vi "Acquisizione statica.vi"() -> ()   [LabVIEW 2017]
uses:
  <vilib>/Analysis/4window.llb/windowTd.ctl
  <vilib>/measure/maspectr.llb/Power Spectrum and PSD Export Mode.ctl
  <vilib>/DAQmx/read.llb/DAQmx Read (Analog 1D Wfm NChan NSamp).vi
  <vilib>/DAQmx/configure/timing.llb/DAQmx Timing (Sample Clock).vi
  <vilib>/DAQmx/miscellaneous.llb/DAQmx Fill In Error Info.vi
  <vilib>/measure/maspectr.llb/FFT Power Spectrum and PSD for N Chan.vi
  <vilib>/measure/maspectr.llb/FFT Spectrum (Mag-Phase) for N Chan.vi
  <vilib>/measure/maspectr.llb/Frequency Response Function (Mag-Phase) N-M.vi
  <vilib>/Waveform/WDTOps.llb/WDT Index Channel DBL.vi
  <vilib>/Waveform/WDTOps.llb/WDT Append Waveforms DBL.vi
  <vilib>/measure/NI_MAPro.lvlib
  <vilib>/Analysis/NI_AALPro.lvlib
panel:
  out "iterazioni":i32
  out "out":bool
  out "error out":errorcluster
  out "salvato":bool
  out "std dev":bool
  out "mean":bool
  out "sample":i32
  in  "std dev max":dbl
  in  "mean/sample max":dbl
  out "mean/sample":dbl
  out "mean":dbl format="%0.2f"
  out "std dev/semple":dbl
  out "standard deviation":dbl format="%0.2f"
  in  "Massa":string="_"
  in  "secondi da salvare":i32=1
  in  "restart averaging (F)":bool
  in  "window":T1 items=["Rectangle"=0, "Hanning"=1, "Hamming"=2, "Blackman-Harris"=3, "Exact Blackman"=4, "Blackman"=5, "Flat Top"=6, "4 Term B-Harris "=7, "7 Term B-Harris"=8, "Low Sidelobe"=9, "Blackman Nuttall"=11, "Triangle"=30, "Bartlett-Hanning"=31, "Bohman"=32, "Parzen"=33, "Welch"=34, "Kaiser"=60, "Dolph-Chebyshev"=61, "Gaussian"=62]
  in  "averaging parameters":T2={"averaging mode"=enum."Vector averaging", "weighting mode"=enum."Linear", "number of averages"=1000}
  in  "Tab Control 2":enum32{"TH", "FRF", "PSD", "FFT"}(tab)
  out "Waveform Chart":waveform(dbl)[](graph)
  out "Waveform Graph":cluster{"f0":dbl, "df":dbl, "magnitude":dbl[]}[](graph)
  in  "REFERENCE CHANNEL":i32=1
  out "Waveform Graph 2":cluster{"f0":dbl, "df":dbl, "magnitude":dbl[]}[](graph)
  out "Magnitude 2":cluster{"f0":dbl, "df":dbl, "magnitude":dbl[]}[](graph)
  out "Magnitude":cluster{"f0":dbl, "df":dbl, "magnitude":dbl[]}[](graph)
  in  "SAVE?":bool
  in  "export":path
  in  "stop":bool
  in  "acquisition":T3={"Fs"=2000.0, "group sample/s"=2000, "generation task"="ModAnalEs"} {"Fs" format="%.2p"}
  # "x10^-3"
  # "x10^-6"
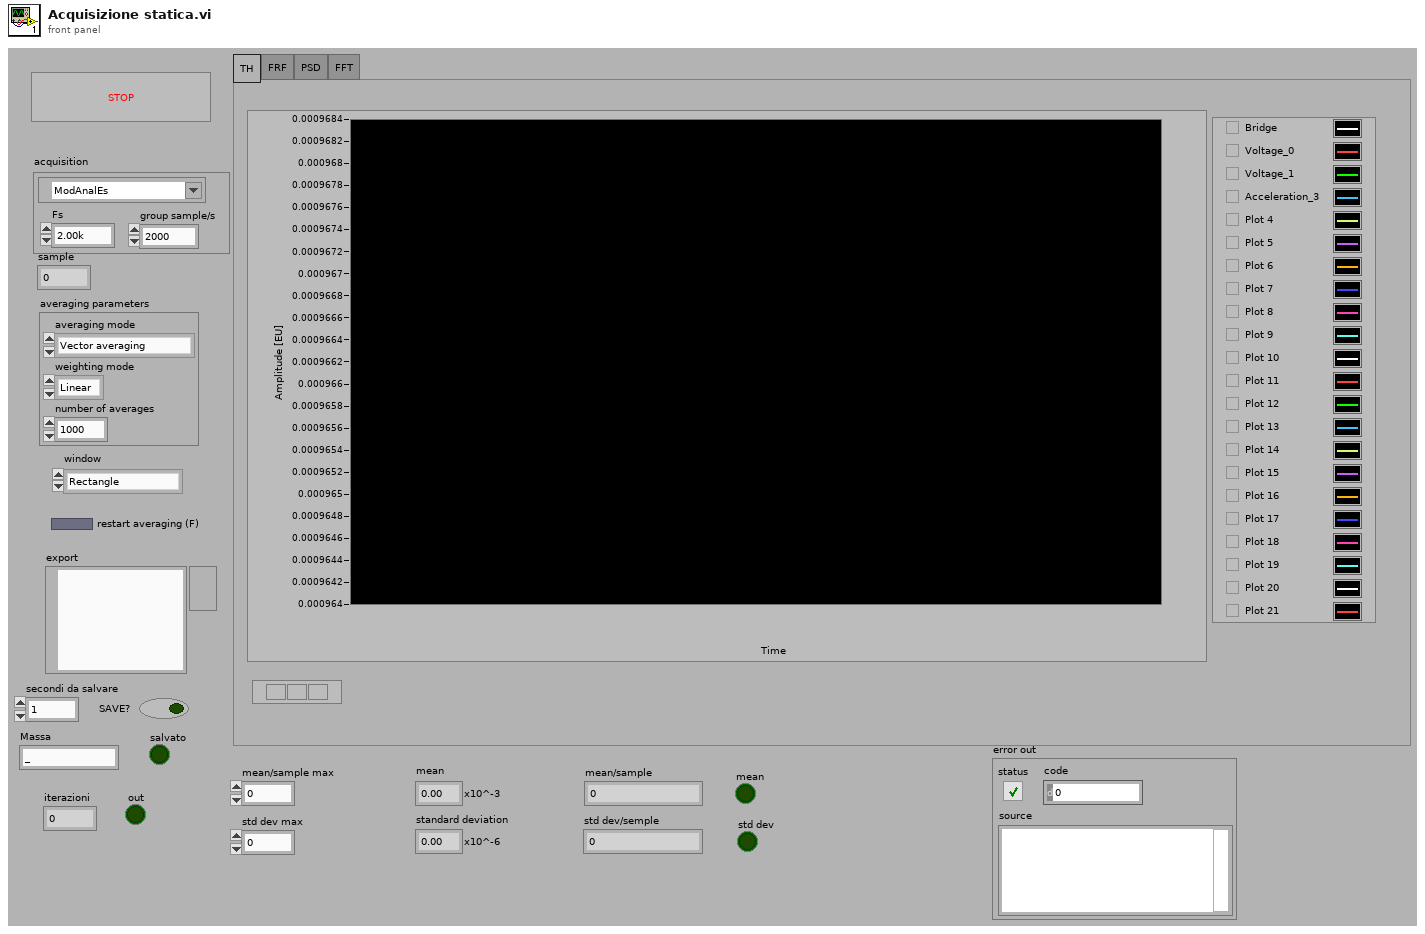
[diagram p1: front panel]
types:
  T1 = typedef "NI_AALPro.lvlib/windowTd.ctl" = u32
  T2 = cluster{"averaging mode":enum16{"No averaging", "Vector averaging", "RMS averaging", "Peak hold"}, "weighting mode":enum16{"Linear", "Exponential"}, "number of averages":u32}
  T3 = cluster{"Fs":dbl, "group sample/s":i32, "generation task":refnum<k21>}
  T4 = cluster{"dB On (F)":bool, "unwrap phase (F)":bool, "convert to degree (F)":bool}
  T5 = typedef "NI_MAPro.lvlib/Power Spectrum and PSD Export Mode.ctl" = u16
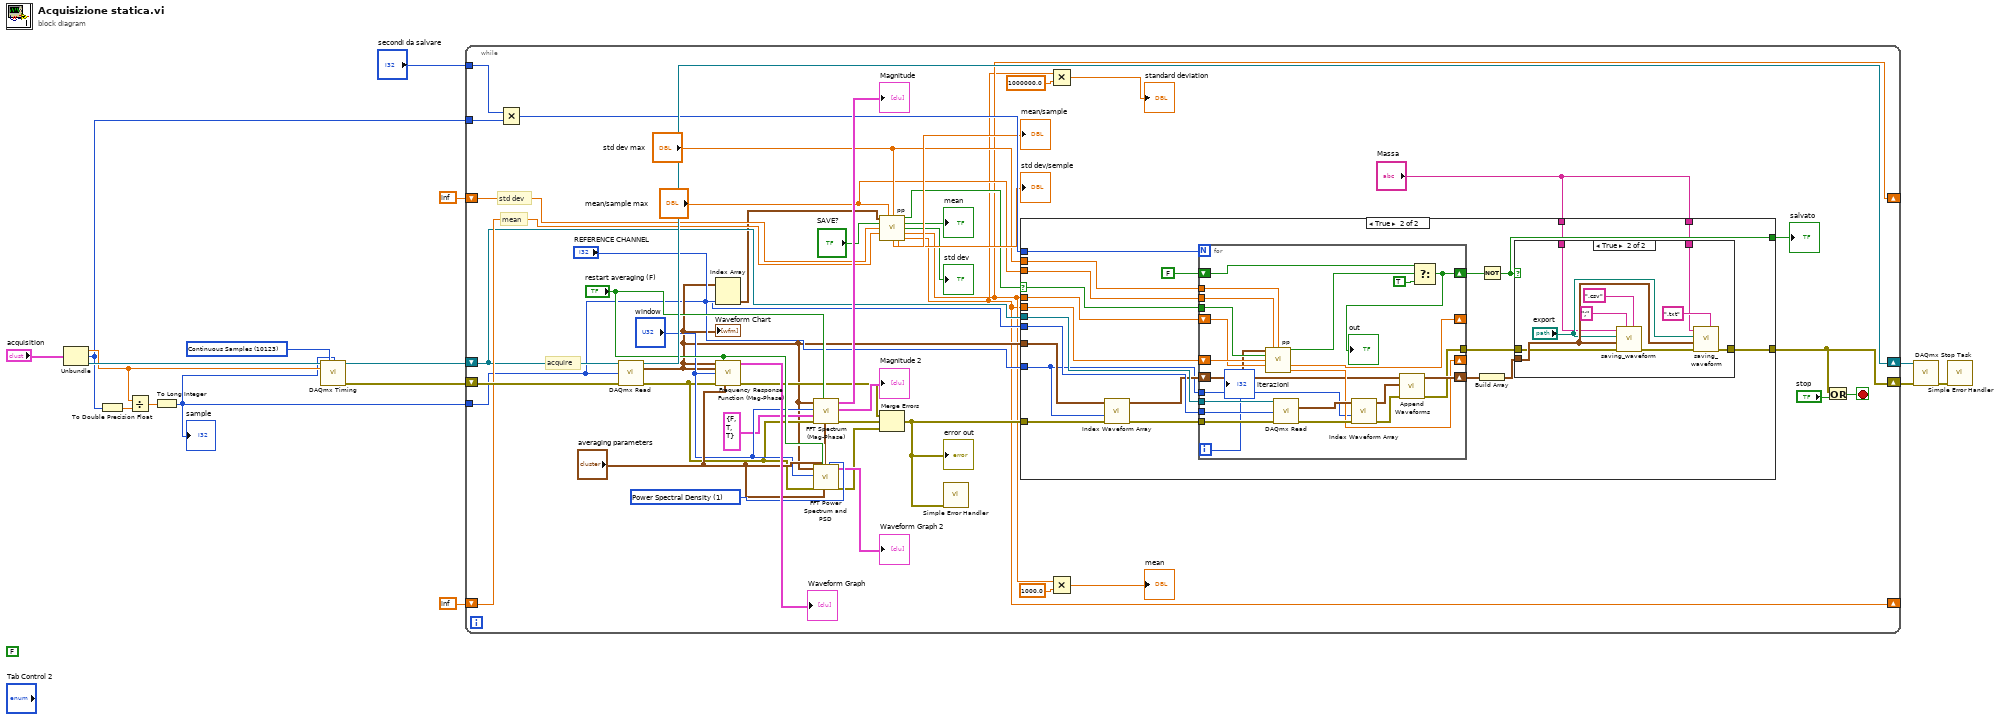
[diagram p0: block diagram]
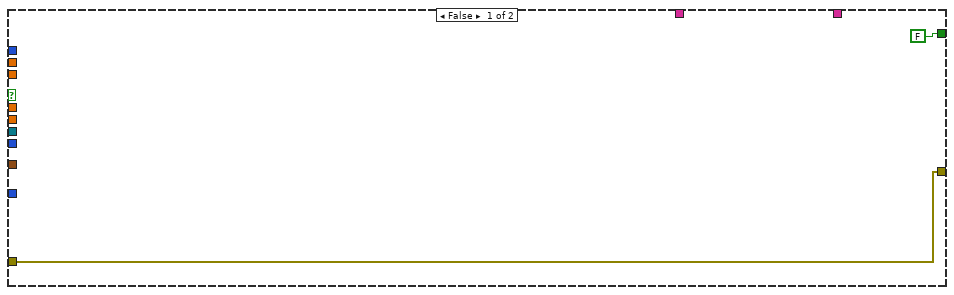
[diagram p2: hidden frame]
diagram:
  (unwired) FALSE
  w12 = 10123 items=["Finite Samples"=10178, "Continuous Samples"=10123, "Hardware Timed Single Point"=12522] ("sample mode")
  n1 = Unbundle("acquisition") -> ("Fs"=w7:dbl, "group sample/s"=w2:i32, "generation task"=w13:refnum<k21>)
  n2 = To Double Precision Float(number=w2) -> (double precision float=w5:dbl)
  n3 = Divide(x=w7, y=w5) -> (x/y=w6:dbl)
  n4 = To Long Integer(number=w6) -> (32bit integer=w1:i32)
  "sample" <- w1
  n5 = call-poly <vilib>:"DAQmx Timing.vi"("task/channels in"=w13, "sample mode"=w12, "samples per channel"=w1, "rate"=w7) -> ("task out"=w11:refnum<k21>, "error out"=w10:errorcluster)  [unwired: 10 in]
  n6 = while {
    shift-right: [w60] -> w15
    shift-left: w11 -> [w45]
    shift-right: [w48] -> w16
    shift-left: w10 -> [w61]
    tunnel: w2 -> [w44]
    shift-right: [w23] -> _
    shift-left: inf -> [w47]
    shift-right: [w19] -> _
    shift-left: inf -> [w46]
    tunnel: "secondi da salvare" -> [w42]
    tunnel: w1 -> [w24]
    stop <- w49 stop-if-true
    w58 = T5 1 items=["Power Spectrum", "Power Spectral Density"] ("export mode")
    # "mean"
    # "std dev"
    # "acquire"
    n7 = Multiply(x=w42, y=w44) -> (x*y=w43:i32)
    n8 = call-poly <vilib>:"DAQmx Read.vi"("task/channels in"=w45, "number of samples per channel"=w24, "error in"=w61) -> ("task out"=w60:refnum<k21>, "data"=w25:waveform(dbl)[], "error out"=w31:errorcluster)  [unwired: 10 in]
    "Waveform Chart" <- w25
    n9 = Index Array(array=w25, index #2="REFERENCE CHANNEL") -> (element #2=w41:waveform(dbl))  [unwired: 1 in, 1 out]
    n10 = call-poly <vilib>:"Frequency Response Function (Mag-Phase).vi"("time signals X"=w25, "restart averaging (F)"="restart averaging (F)", "time signals Y"=w25, "window"="window", "error in (no error)"=w31, "averaging parameters"="averaging parameters") -> ("magnitudes"=→"Waveform Graph":cluster{"f0":dbl, "df":dbl, "magnitude":dbl[]}[], "error out"=w28:errorcluster)  [unwired: 4 in, 4 out]
    n11 = call-poly <vilib>:"FFT Power Spectrum and PSD.vi"("export mode"=w58, "averaging parameters"="averaging parameters", "restart averaging (F)"="restart averaging (F)", "error in (no error)"=w31, "window"="window", "time signals"=w25) -> ("error out"=w30:errorcluster, "Power Spectrum / PSD"=→"Waveform Graph 2":cluster{"f0":dbl, "df":dbl, "magnitude":dbl[]}[])  [unwired: 2 in, 2 out]
    n12 = call-poly <vilib>:"FFT Spectrum (Mag-Phase).vi"("averaging parameters"="averaging parameters", "restart averaging (F)"="restart averaging (F)", "error in (no error)"=w31, "view"=T4 {"dB On (F)"=FALSE, "unwrap phase (F)"=TRUE, "convert to degree (F)"=TRUE}, "window"="window", "time signals"=w25) -> ("error out"=w29:errorcluster, "phases"=→"Magnitude 2":cluster{"f0":dbl, "df":dbl, "phase":dbl[]}[], "magnitudes"=→"Magnitude":cluster{"f0":dbl, "df":dbl, "magnitude":dbl[]}[])  [unwired: 1 in, 2 out]
    n13 = call "pp.vi"("Waveform"=w41, "mean/sample max"="mean/sample max", "std dev max"="std dev max", "SAVE?"="SAVE?", "prev std dev"=w47, "prev mean"=w46) -> ("out"=w37:bool, 6:"mean"=→"mean":bool, "std dev"=→"std dev":bool, 10:"mean"=w23:dbl, "std dev/semple"=→"std dev/semple":dbl, "mean/sample"=→"mean/sample":dbl, "standard deviation"=w19:dbl)  [unwired: 3 in]
    n14 = Merge Errors(w28, w29, w30) -> (w26:errorcluster)
    "error out" <- w26
    n15 = call <vilib>:"Simple Error Handler.vi"("error in (no error)"=w26) -> ()  [unwired: 4 in, 5 out]
    n16 = case shown="True" w37 {
      selector: w37 -> [_ w78]
      tunnel: w26 -> [w63 w67]
      tunnel: [w63 w85] -> w48
      tunnel: w25 -> [_ w70]
      tunnel: w43 -> [_ w84]
      tunnel: w45 -> [_ w83]
      tunnel: w24 -> [_ w81]
      tunnel: w19 -> [_ w77]
      tunnel: w23 -> [_ w76]
      tunnel: "std dev max" -> [_ w75]
      tunnel: "mean/sample max" -> [_ w74]
      tunnel: [FALSE w71] -> w32
      tunnel: "REFERENCE CHANNEL" -> [_ w68]
      tunnel: "Massa" -> [_ w65]
      tunnel: "Massa" -> [_ w64]
      frame False {
      }
      frame True {
        n17 = call-poly <vilib>:"Index Waveform Array.vi"("error in (no error)"=w67, "index"=w68, "waveform array"=w70) -> ("error out"=w66:errorcluster, "waveform"=w69:waveform(dbl))  [unwired: 7 in]
        n18 = for {
          N: w84 -> [_]
          shift-right: [w108] -> w80
          shift-left: w69 -> [w88]
          tunnel: [w103] -> w82
          tunnel: w66 -> [w102]
          tunnel: w83 -> [w101]
          tunnel: w81 -> [w100]
          tunnel: w78 -> [w99]
          shift-right: [w95] -> _
          shift-left: w77 -> [w98]
          shift-right: [w96] -> _
          shift-left: w76 -> [w97]
          tunnel: w75 -> [w94]
          tunnel: w74 -> [w93]
          shift-right: [w86] -> w72
          shift-left: FALSE -> [w91]
          tunnel: w68 -> [w89]
          i -> [w87]
          n19 = call "pp.vi"("Waveform"=w88, "mean/sample max"=w93, "std dev max"=w94, "SAVE?"=w99, "prev std dev"=w98, "prev mean"=w97) -> ("out"=w92:bool, "mean"=w96:dbl, "standard deviation"=w95:dbl)  [unwired: 3 in, 4 out]
          n20 = call-poly <vilib>:"DAQmx Read.vi"("task/channels in"=w101, "number of samples per channel"=w100, "error in"=w102) -> ("data"=w107:waveform(dbl)[], "error out"=w105:errorcluster)  [unwired: 10 in, 1 out]
          n21 = call-poly <vilib>:"Index Waveform Array.vi"("error in (no error)"=w105, "index"=w89, "waveform array"=w107) -> ("error out"=w104:errorcluster, "waveform"=w106:waveform(dbl))  [unwired: 7 in]
          n22 = call-poly <vilib>:"Append Waveforms.vi"("error in (no error)"=w104, "waveform B"=w106, "waveform A"=w88) -> ("error out"=w103:errorcluster, "waveform out"=w108:waveform(dbl))  [unwired: 7 in]
          n23 = Select(t=w91, s=w92, f=TRUE) -> (s? t:f=w86:bool)
          "out" <- w86
          "iterazioni" <- w87
        }
        n24 = Not(x=w72) -> (.not. x?=w71:bool)
        n25 = Build Array(w80) -> (w79:waveform(dbl)[])
        n26 = case shown="True" w71 {
          tunnel: w79 -> [_ w117]
          tunnel: [w109 w113] -> w85
          tunnel: w82 -> [w109 w112]
          tunnel: w65 -> [_ w111]
          tunnel: w64 -> [_ w110]
          frame False {
          }
          frame True {
            n27 = call "saving_waveform.vi"("extension"=".csv", "delimiter (Tab)"=";", "error in (no error)"=w112, "Array"=w117, "directory"="export", "Massa"=w110) -> ("error out"=w114:errorcluster)  [unwired: 5 in]
            n28 = call "saving_waveform.vi"("extension"=".txt", "error in (no error)"=w114, "Array"=w117, "directory"="export", "Massa"=w111) -> ("error out"=w113:errorcluster)  [unwired: 6 in]
          }
        }
      }
    }
    "salvato" <- w32
    n29 = Multiply(x=w19, y=1000000.0) -> (x*y=→"standard deviation":dbl)
    n30 = Multiply(x=w23, y=1000.0) -> (x*y=→"mean":dbl)
    n31 = Or(x=w48, y="stop") -> (x .or. y?=w49:bool)
  }
  n32 = call <vilib>:"DAQmx Stop Task.vi"("task/channels in"=w15, "error in"=w16) -> ("error out"=w9:errorcluster)  [unwired: 12 in, 1 out]
  n33 = call <vilib>:"Simple Error Handler.vi"("error in (no error)"=w9) -> ()  [unwired: 4 in, 5 out]
